vi "init.vi"() -> (0 "error":errorcluster, 3 "input cluster":T1)   [LabVIEW 2025]
uses:
  Classes/controller/controller.lvclass
  Classes/hardware/hardware.lvclass
  <vilib>/Utility/sysdir.llb/System Directory Type.ctl
  76d21f72-6cd7-488b-a7de-b4377f31087f.vi
  <vilib>/JDP Science/JSONtext/JSON text to Variant.vi
  <vilib>/JDP Science/JSONtext/LVClass Serializer/JSONtext LVClass Serializer.lvclass
  Classes/data log/data log.lvclass
panel:
  in  "Relay Inputs":bool[](array[boolean])
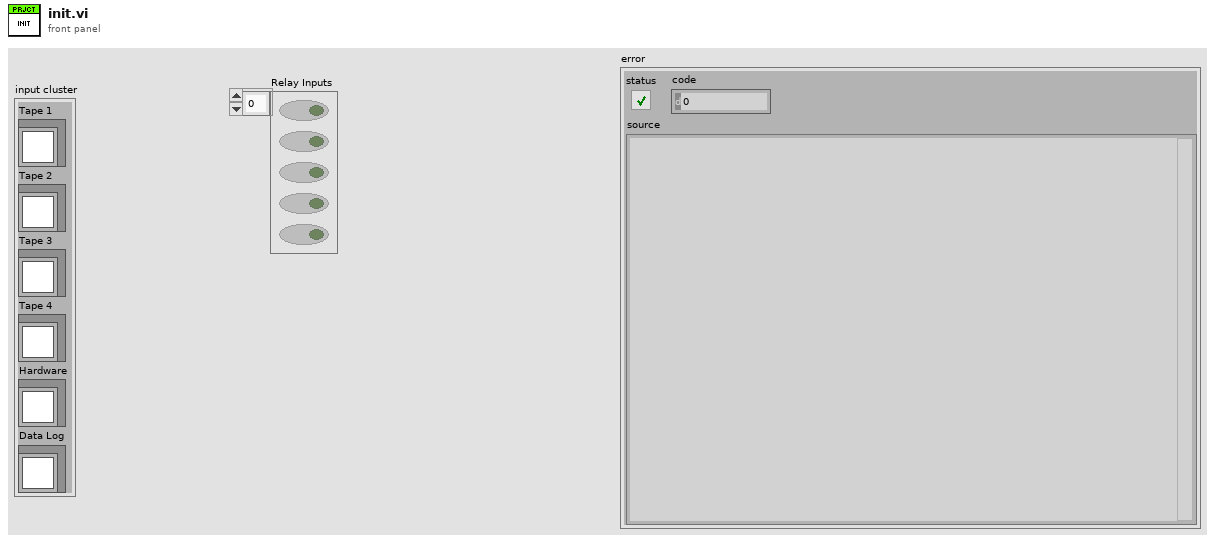
[diagram p1: front panel]
types:
  T1 = cluster{"Tape 1":refnum<class "controller.lvclass">, "Tape 2":refnum<class "controller.lvclass">, "Tape 3":refnum<class "controller.lvclass">, "Tape 4":refnum<class "controller.lvclass">, "Hardware":refnum<class "hardware.lvclass">, "Data Log":refnum<class "data log.lvclass">}
  T2 = cluster{"Tape_1":refnum<class "controller.lvclass">, "Tape_2":refnum<class "controller.lvclass">, "Tape_3":refnum<class "controller.lvclass">, "Tape_4":refnum<class "controller.lvclass">, "Hardware":refnum<class "hardware.lvclass">, "Data_Log":refnum<class "data log.lvclass">}
  T3 = cluster{"Tape_1":cluster{"PID_gains":cluster{"P":dbl, "I":dbl, "D":dbl}, "PID_prev":cluster{"e_prev":dbl, "e_int":dbl}, "Index":i32}, "Tape_2":cluster{"PID_gains":cluster{"P":dbl, "I":dbl, "D":dbl}, "PID_prev":cluster{"e_prev":dbl, "e_int":dbl}, "Index":i32}, "Tape_3":cluster{"PID_gains":cluster{"P":dbl, "I":dbl, "D":dbl}, "PID_prev":cluster{"e_prev":dbl, "e_int":dbl}, "Index":i32}, "Tape_4":cluster{"PID_gains":cluster{"P":dbl, "I":dbl, "D":dbl}, "PID_prev":cluster{"e_prev":dbl, "e_int":dbl}, "Index":i32}}
  T4 = typedef "System Directory Type.ctl" = i32
  T5 = cluster{"PID_gains":cluster{"P":dbl, "I":dbl, "D":dbl}, "PID_prev":cluster{"e_prev":dbl, "e_int":dbl}, "Index":i32}
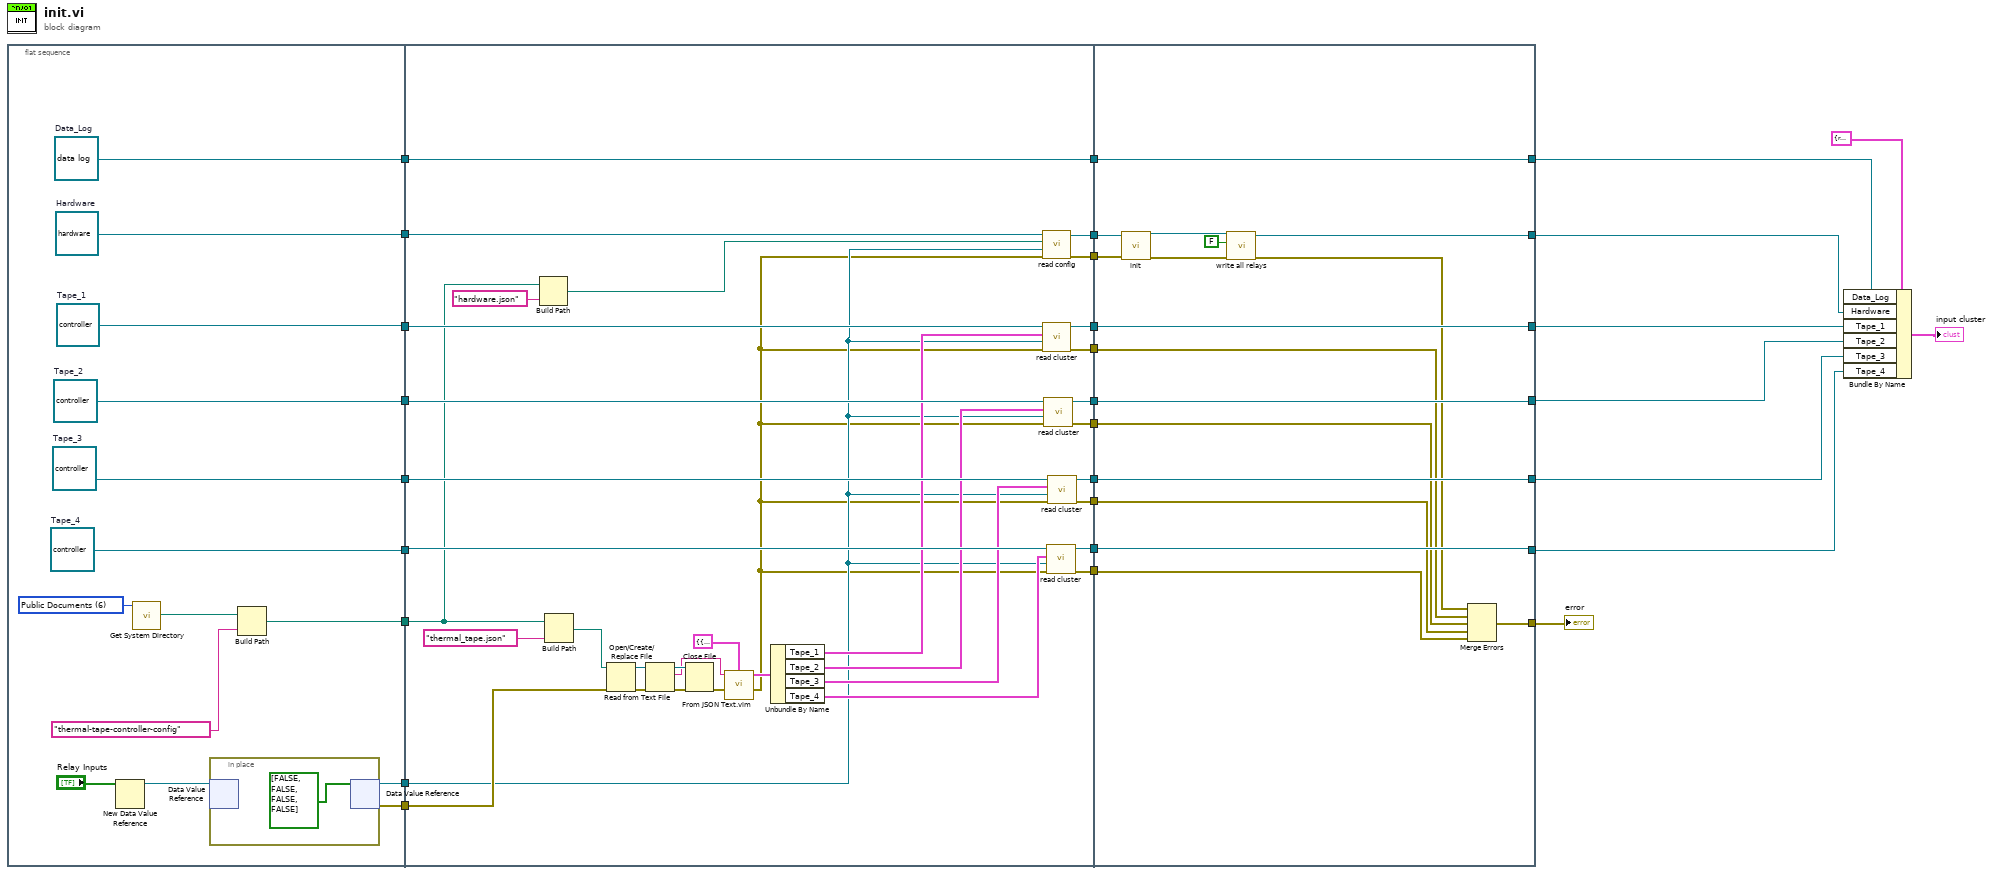
[diagram p0: block diagram]
diagram:
  n1 = flat-sequence {
    tunnel: [w43] -> w25
    tunnel: [w42] -> w24
    tunnel: [w41] -> w23
    tunnel: [w40] -> w22
    tunnel: [w36] -> w20
    tunnel: [w33] -> w10
    tunnel: [w32] -> w9
    tunnel: [w31] -> w8
    tunnel: [w30] -> w4
    tunnel: w25 -> [w63]
    tunnel: w24 -> [w62]
    tunnel: w23 -> [w61]
    tunnel: w22 -> [w60]
    tunnel: w20 -> [w53]
    tunnel: [w71] -> w18
    tunnel: [w70] -> w17
    tunnel: [w69] -> w16
    tunnel: [w68] -> w15
    tunnel: [w67] -> w14
    tunnel: [w66] -> w13
    tunnel: [w65] -> w12
    tunnel: [w64] -> w11
    tunnel: w10 -> [w55]
    tunnel: w9 -> [w51]
    tunnel: w8 -> [w49]
    tunnel: [w47] -> w7
    tunnel: [w46] -> w6
    tunnel: w4 -> [w45]
    tunnel: [w45] -> w3
    tunnel: [w97] -> w21
    tunnel: [w94] -> w26
    tunnel: [w95] -> w27
    tunnel: [w96] -> w28
    tunnel: [w89] -> w19
    tunnel: w18 -> [w97]
    tunnel: w17 -> [w94]
    tunnel: w16 -> [w92]
    tunnel: w15 -> [w93]
    tunnel: w14 -> [w95]
    tunnel: w13 -> [w91]
    tunnel: w12 -> [w96]
    tunnel: w11 -> [w90]
    tunnel: w7 -> [w88]
    tunnel: w6 -> [w87]
    tunnel: [w82] -> w5
    tunnel: w3 -> [w81]
    tunnel: [w81] -> w2
    frame #0 {
      w30 = refnum<class "data log.lvclass"> refnum  # Data_Log
      w31 = refnum<class "hardware.lvclass"> refnum  # Hardware
      w39 = T4 6 items=["User Home"=0, "User Desktop"=1, "User Documents"=2, "User Application Data"=3, "User Preferences"=4, "User Temporary"=5, "Public Documents"=6, "Public Application Data"=7, "Public Preferences"=8, "Public Cache"=13, "System Core Libraries"=9, "System Installed Libraries"=10, "Application Files"=11, "Boot Volume Root"=12] ("system directory type")
      w43 = refnum<class "controller.lvclass"> refnum  # Tape_4
      w42 = refnum<class "controller.lvclass"> refnum  # Tape_3
      w41 = refnum<class "controller.lvclass"> refnum  # Tape_2
      w40 = refnum<class "controller.lvclass"> refnum  # Tape_1
      n2 = New Data Value Reference(data value="Relay Inputs") -> (data value reference=w34:refnum<data-value>)  [unwired: 1 in, 1 out]
      n3 = call <vilib>:"Get System Directory.vi"("system directory type"=w39) -> ("system directory"=w38:path)  [unwired: 10 in]
      n4 = in-place {
        n5 = in-place-dvr #1(w34) -> ()  [unwired: 2 out]
        n6 = in-place-dvr #1(bool[] [FALSE, FALSE, FALSE, FALSE] ("data")) -> (w32:refnum<data-value>, w33:errorcluster)
      }
      n7 = Build Path(base path=w38, name or relative path="thermal-tape-controller-config") -> (appended path=w36:path)
    }
    frame #1 {
      n8 = Build Path(base path=w53, name or relative path="hardware.json") -> (appended path=w50:path)
      n9 = Build Path(base path=w53, name or relative path="thermal_tape.json") -> (appended path=w54:path)
      n10 = Open/Create/Replace File(file path (use dialog)=w54, error in=w55) -> (refnum out=w76:refnum<file>, error out=w79:errorcluster)  [unwired: 4 in, 1 out]
      n11 = Read from Text File(file (use dialog)=w76, error in=w79) -> (refnum out=w77:refnum<file>, text=w75:string, error out=w78:errorcluster)  [unwired: 2 in, 1 out]
      n12 = Close File(refnum=w77, error in=w78) -> (error out=w74:errorcluster)  [unwired: 1 out]
      n13 = call "From JSON Text.vim"("Data Type and Default Value"=T3 {"Tape_1"={"PID_gains"={"P"=0.0, "I"=0.0, "D"=0.0}, "PID_prev"={"e_prev"=0.0, "e_int"=0.0}, "Index"=0}, "Tape_2"={"PID_gains"={"P"=0.0, "I"=0.0, "D"=0.0}, "PID_prev"={"e_prev"=0.0, "e_int"=0.0}, "Index"=0}, "Tape_3"={"PID_gains"={"P"=0.0, "I"=0.0, "D"=0.0}, "PID_prev"={"e_prev"=0.0, "e_int"=0.0}, "Index"=0}, "Tape_4"={"PID_gains"={"P"=0.0, "I"=0.0, "D"=0.0}, "PID_prev"={"e_prev"=0.0, "e_int"=0.0}, "Index"=0}}, "error in (no error)"=w74, "JSON"=w75) -> ("error out"=w48:errorcluster, "Data out"=w72:T3)  [unwired: 7 in]
      n14 = Unbundle By Name(w72) -> ("Tape_1"=w59:T5, "Tape_2"=w58:T5, "Tape_3"=w57:T5, "Tape_4"=w56:T5)
      n15 = call-dynamic "read config.vi"("error in (no error)"=w48, "data value reference"=w51, "file path (use dialog)"=w50, "hardware in"=w49) -> ("error out"=w46:errorcluster, "hardware out"=w47:refnum<class "hardware.lvclass">)  [unwired: 6 in]
      n16 = call-dynamic "read cluster.vi"("error in (no error)"=w48, "data value reference"=w51, "Tape Cluster"=w59, "controller in"=w60) -> ("error out"=w68:errorcluster, "controller out"=w71:refnum<class "controller.lvclass">)  [unwired: 6 in]
      n17 = call-dynamic "read cluster.vi"("error in (no error)"=w48, "data value reference"=w51, "Tape Cluster"=w58, "controller in"=w61) -> ("error out"=w69:errorcluster, "controller out"=w70:refnum<class "controller.lvclass">)  [unwired: 6 in]
      n18 = call-dynamic "read cluster.vi"("error in (no error)"=w48, "data value reference"=w51, "Tape Cluster"=w56, "controller in"=w63) -> ("error out"=w64:errorcluster, "controller out"=w65:refnum<class "controller.lvclass">)  [unwired: 6 in]
      n19 = call-dynamic "read cluster.vi"("error in (no error)"=w48, "data value reference"=w51, "Tape Cluster"=w57, "controller in"=w62) -> ("error out"=w66:errorcluster, "controller out"=w67:refnum<class "controller.lvclass">)  [unwired: 6 in]
    }
    frame #2 {
      n20 = call-dynamic "init.vi"("error in (no error)"=w87, "hardware in"=w88) -> ("error out"=w85:errorcluster, "hardware out"=w86:refnum<class "hardware.lvclass">)  [unwired: 8 in]
      n21 = call-dynamic "write all relays.vi"("error in (no error)"=w85, "Boolean"=FALSE, "hardware in"=w86) -> ("error out"=w83:errorcluster, "hardware out"=w82:refnum<class "hardware.lvclass">)  [unwired: 7 in]
      n22 = Merge Errors(w83, w93, w92, w91, w90) -> (w89:errorcluster)
    }
  }
  n23 = Bundle By Name(cluster=T2 {"Tape_1"=refnum, "Tape_2"=refnum, "Tape_3"=refnum, "Tape_4"=refnum, "Hardware"=refnum, "Data_Log"=refnum} ("input cluster"), "Data_Log"=w2, "Hardware"=w5, "Tape_1"=w21, "Tape_2"=w26, "Tape_3"=w27, "Tape_4"=w28) -> (→"input cluster":T2)
  "error" <- w19
